vi "Initialize Default.vi"(8 "error in (no error)":errorcluster, 11 "UDP Thread Configuration in":refnum<class "UDP Thread Configuration.lvclass">) -> (0 "error out":errorcluster, 3 "UDP Thread Configuration out":refnum<class "UDP Thread Configuration.lvclass">)   [LabVIEW 2017, in "DSF Core.lvlib" / "UDP Thread Configuration.lvclass"]
uses:
  UDP Thread Configuration.lvclass
  Classes/Configuration/Configuration.lvclass
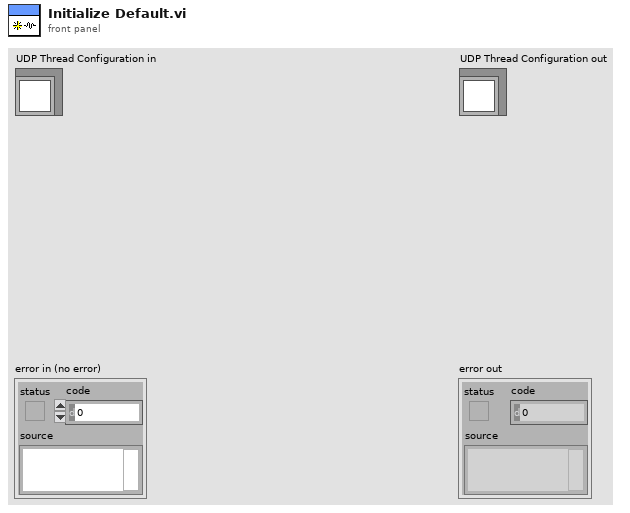
[diagram p1: front panel]
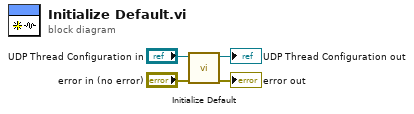
[diagram p0: block diagram]
diagram:
  n1 = call-parent "Initialize Default.vi"("error in (no error)"="error in (no error)", "Configuration in"="UDP Thread Configuration in") -> ("error out"=→"error out":errorcluster, "Configuration out"=→"UDP Thread Configuration out":refnum<class "UDP Thread Configuration.lvclass">)  [unwired: 8 in]
